vi "example_02_convert.vi"() -> ()   [LabVIEW 2015, in "lv-unit-conversion.lvlib"] (continued)
 gallon per minute foot", "dimension"="L2/T", "is_si_unit"=TRUE, "category"="derived", "base_unit"="m3/(s.m)", "conversion_reference"="DERIVED", "is_exact"=TRUE, "a"=0.0, "b"=0.003785411784, "c"=18.288, "d"=0.0, "underlying_def"="", "description"=""}, {"symbol"="m3/(d.m)", "name"="(cubic metre per day) per metre", "dimension"="L2/T", "is_si_unit"=TRUE, "category"="derived", "base_unit"="m3/(s.m)", "conversion_reference"="DERIVED", "is_exact"=TRUE, "a"=0.0, "b"=1.0, "c"=86400.0, "d"=0.0, "underlying_def"="", "description"=""}, {"symbol"="m3/(h.m)", "name"="(cubic metre per hour) per metre", "dimension"="L2/T", "is_si_unit"=TRUE, "category"="derived", "base_unit"="m3/(s.m)", "conversion_reference"="DERIVED", "is_exact"=TRUE, "a"=0.0, "b"=1.0, "c"=3600.0, "d"=0.0, "underlying_def"="", "description"=""}, {"symbol"="m3/(s.ft)", "name"="(cubic metre per second) per foot", "dimension"="L2/T", "is_si_unit"=TRUE, "category"="derived", "base_unit"="m3/(s.m)", "conversion_reference"="DERIVED", "is_exact"=TRUE, "a"=0.0, "b"=1.0, "c"=0.3048, "d"=0.0, "underlying_def"="", "description"=""}, {"symbol"="cSt", "name"="centistokes", "dimension"="L2/T", "is_si_unit"=TRUE, "category"="prefixed", "base_unit"="m2/s", "conversion_reference"="DERIVED", "is_exact"=TRUE, "a"=0.0, "b"=1e-06, "c"=1.0, "d"=0.0, "underlying_def"="", "description"=""}, {"symbol"="rd", "name"="rad", "dimension"="L2/T2", "is_si_unit"=TRUE, "category"="atom", "base_unit"="Gy", "conversion_reference"="NIST-SI", "is_exact"=TRUE, "a"=0.0, "b"=0.01, "c"=1.0, "d"=0.0, "underlying_def"="1/100 Gy", "description"="A obsolete unit of absorbed radiation dose. \n\t\t\t\tIt was originally defined in CGS units in 1953 as the dose causing 100 ergs of energy to be absorbed \n\t\t\t\tby one gram of matter. \n\t\t\t\tIt has been replaced by the gray in most of the world.\n\t\t\t"}, {"symbol"="Gy", "name"="gray", "dimension"="L2/T2", "is_si_unit"=TRUE, "category"="atom-special", "base_unit"="", "conversion_reference"="", "is_exact"=FALSE, "a"=0.0, "b"=0.0, "c"=0.0, "d"=0.0, "underlying_def"="J/kg", "description"="The absorbed dose when the energy per unit mass imparted to matter by ionizing radiation is 1 J/kg"}, {"symbol"="Sv", "name"="sievert", "dimension"="L2/T2", "is_si_unit"=TRUE, "category"="atom-special", "base_unit"="", "conversion_reference"="", "is_exact"=FALSE, "a"=0.0, "b"=0.0, "c"=0.0, "d"=0.0, "underlying_def"="J/kg", "description"="The dose equivalent when the absorbed dose of ionizing radiation multiplied by the dimensionless \n\t\t\t\tfactors Q (quality factor) and N (product of any of the multiplying factors) stipulated by the \n\t\t\t\tInternational Commission on Radiological Protection is 1.0 J/kg.\n\t\t\t"}, {"symbol"="rem", "name"="rem", "dimension"="L2/T2", "is_si_unit"=TRUE, "category"="atom-allowed", "base_unit"="Sv", "conversion_reference"="NIST-SI", "is_exact"=TRUE, "a"=0.0, "b"=0.01, "c"=1.0, "d"=0.0, "underlying_def"="1/100 Sv", "description"="A unit of radiation dosage (such as from X rays) applied to humans. \n\t\t\t\tDerived from the phrase Roentgen equivalent man, the rem is now defined as the dosage in rads that \n\t\t\t\twill cause the same amount of biological injury as one rad of X rays or gamma rays.\n\t\t\t"}, {"symbol"="J/kg", "name"="joule per kilogram", "dimension"="L2/T2", "is_si_unit"=TRUE, "category"="derived", "base_unit"="", "conversion_reference"="", "is_exact"=FALSE, "a"=0.0, "b"=0.0, "c"=0.0, "d"=0.0, "underlying_def"="", "description"=""}, {"symbol"="Btu[IT]/lbm", "name"="BTU per pound-mass", "dimension"="L2/T2", "is_si_unit"=TRUE, "category"="derived", "base_unit"="J/kg", "conversion_reference"="DERIVED", "is_exact"=TRUE, "a"=0.0, "b"=2326.0, "c"=1.0, "d"=0.0, "underlying_def"="", "description"=""}, {"symbol"="cal[th]/g", "name"="calorie per gram", "dimension"="L2/T2", "is_si_unit"=TRUE, "category"="derived", "base_unit"="J/kg", "conversion_reference"="DERIVED", "is_exact"=TRUE, "a"=0.0, "b"=4184.0, "c"=1.0, "d"=0.0, "underlying_def"="", "description"=""}, {"symbol"="cal[th]/kg", "name"="calorie per kilogram", "dimension"="L2/T2", "is_si_unit"=TRUE, "category"="derived", "base_unit"="J/kg", "conversion_reference"="DERIVED", "is_exact"=TRUE, "a"=0.0, "b"=4.184, "c"=1.0, "d"=0.0, "underlying_def"="", "description"=""}, {"symbol"="cal[th]/lbm", "name"="calorie per pound-mass", "dimension"="L2/T2", "is_si_unit"=TRUE, "category"="derived", "base_unit"="J/kg", "conversion_reference"="DERIVED", "is_exact"=TRUE, "a"=0.0, "b"=4.184, "c"=0.45359237, "d"=0.0, "underlying_def"="", "description"=""}, {"symbol"="erg/g", "name"="erg per gram", "dimension"="L2/T2", "is_si_unit"=TRUE, "category"="derived", "base_unit"="J/kg", "conversion_reference"="DERIVED", "is_exact"=TRUE, "a"=0.0, "b"=0.0001, "c"=1.0, "d"=0.0, "underlying_def"="", "description"=""}, {"symbol"="erg/kg", "name"="erg per kilogram", "dimension"="L2/T2", "is_si_unit"=TRUE, "category"="derived", "base_unit"="J/kg", "conversion_reference"="DERIVED", "is_exact"=TRUE, "a"=0.0, "b"=1e-07, "c"=1.0, "d"=0.0, "underlying_def"="", "description"=""}, {"symbol"="hp.h/lbm", "name"="horsepower hour per pound-mass", "dimension"="L2/T2", "is_si_unit"=TRUE, "category"="derived", "base_unit"="J/kg", "conversion_reference"="DERIVED", "is_exact"=TRUE, "a"=0.0, "b"=2684519.537696173, "c"=0.45359237, "d"=0.0, "underlying_def"="", "description"=""}, {"symbol"="J/g", "name"="joule per gram", "dimension"="L2/T2", "is_si_unit"=TRUE, "category"="derived", "base_unit"="J/kg", "conversion_reference"="DERIVED", "is_exact"=TRUE, "a"=0.0, "b"=1000.0, "c"=1.0, "d"=0.0, "underlying_def"="", "description"=""}, {"symbol"="kcal[th]/g", "name"="thousand calorie per gram", "dimension"="L2/T2", "is_si_unit"=TRUE, "category"="derived", "base_unit"="J/kg", "conversion_reference"="DERIVED", "is_exact"=TRUE, "a"=0.0, "b"=4184000.0, "c"=1.0, "d"=0.0, "underlying_def"="", "description"=""}, {"symbol"="kcal[th]/kg", "name"="thousand calorie per kilogram", "dimension"="L2/T2", "is_si_unit"=TRUE, "category"="derived", "base_unit"="J/kg", "conversion_reference"="DERIVED", "is_exact"=TRUE, "a"=0.0, "b"=4184.0, "c"=1.0, "d"=0.0, "underlying_def"="", "description"=""}, {"symbol"="kJ/kg", "name"="kilojoule per kilogram", "dimension"="L2/T2", "is_si_unit"=TRUE, "category"="derived", "base_unit"="J/kg", "conversion_reference"="DERIVED", "is_exact"=TRUE, "a"=0.0, "b"=1000.0, "c"=1.0, "d"=0.0, "underlying_def"="", "description"=""}, {"symbol"="kW.h/kg", "name"="kilowatt hour per kilogram", "dimension"="L2/T2", "is_si_unit"=TRUE, "category"="derived", "base_unit"="J/kg", "conversion_reference"="DERIVED", "is_exact"=TRUE, "a"=0.0, "b"=3600000.0, "c"=1.0, "d"=0.0, "underlying_def"="", "description"=""}, {"symbol"="lbf.ft/lbm", "name"="foot pound-force per pound-mass", "dimension"="L2/T2", "is_si_unit"=TRUE, "category"="derived", "base_unit"="J/kg", "conversion_reference"="DERIVED", "is_exact"=TRUE, "a"=0.0, "b"=1.3558179483314003, "c"=0.45359237, "d"=0.0, "underlying_def"="", "description"=""}, {"symbol"="MJ/kg", "name"="megajoule per kilogram", "dimension"="L2/T2", "is_si_unit"=TRUE, "category"="derived", "base_unit"="J/kg", "conversion_reference"="DERIVED", "is_exact"=TRUE, "a"=0.0, "b"=1000000.0, "c"=1.0, "d"=0.0, "underlying_def"="", "description"=""}, {"symbol"="MW.h/kg", "name"="megawatt hour per kilogram", "dimension"="L2/T2", "is_si_unit"=TRUE, "category"="derived", "base_unit"="J/kg", "conversion_reference"="DERIVED", "is_exact"=TRUE, "a"=0.0, "b"=3600000000.0, "c"=1.0, "d"=0.0, "underlying_def"="", "description"=""}, {"symbol"="cGy", "name"="centigray", "dimension"="L2/T2", "is_si_unit"=TRUE, "category"="prefixed", "base_unit"="Gy", "conversion_reference"="DERIVED", "is_exact"=TRUE, "a"=0.0, "b"=0.01, "c"=1.0, "d"=0.0, "underlying_def"="", "description"=""}, {"symbol"="crd", "name"="hundredth of rad", "dimension"="L2/T2", "is_si_unit"=TRUE, "category"="prefixed", "base_unit"="Gy", "conversion_reference"="DERIVED", "is_exact"=TRUE, "a"=0.0, "b"=0.0001, "c"=1.0, "d"=0.0, "underlying_def"="", "description"=""}, {"symbol"="dGy", "name"="decigray", "dimension"="L2/T2", "is_si_unit"=TRUE, "category"="prefixed", "base_unit"="Gy", "conversion_reference"="DERIVED", "is_exact"=TRUE, "a"=0.0, "b"=0.1, "c"=1.0, "d"=0.0, "underlying_def"="", "description"=""}, {"symbol"="drd", "name"="tenth of rad", "dimension"="L2/T2", "is_si_unit"=TRUE, "category"="prefixed", "base_unit"="Gy", "conversion_reference"="DERIVED", "is_exact"=TRUE, "a"=0.0, "b"=0.001, "c"=1.0, "d"=0.0, "underlying_def"="", "description"=""}, {"symbol"="EGy", "name"="exagray", "dimension"="L2/T2", "is_si_unit"=TRUE, "category"="prefixed", "base_unit"="Gy", "conversion_reference"="DERIVED", "is_exact"=TRUE, "a"=0.0, "b"=1e+18, "c"=1.0, "d"=0.0, "underlying_def"="", "description"=""}, {"symbol"="Erd", "name"="million million million rad", "dimension"="L2/T2", "is_si_unit"=TRUE, "category"="prefixed", "base_unit"="Gy", "conversion_reference"="DERIVED", "is_exact"=TRUE, "a"=0.0, "b"=1e+16, "c"=1.0, "d"=0.0, "underlying_def"="", "description"=""}, {"symbol"="fGy", "name"="femtogray", "dimension"="L2/T2", "is_si_unit"=TRUE, "category"="prefixed", "base_unit"="Gy", "conversion_reference"="DERIVED", "is_exact"=TRUE, "a"=0.0, "b"=1e-15, "c"=1.0, "d"=0.0, "underlying_def"="", "description"=""}, {"symbol"="frd", "name"="femtorad", "dimension"="L2/T2", "is_si_unit"=TRUE, "category"="prefixed", "base_unit"="Gy", "conversion_reference"="DERIVED", "is_exact"=TRUE, "a"=0.0, "b"=1e-17, "c"=1.0, "d"=0.0, "underlying_def"="", "description"=""}, {"symbol"="GGy", "name"="gigagray", "dimension"="L2/T2", "is_si_unit"=TRUE, "category"="prefixed", "base_unit"="Gy", "conversion_reference"="DERIVED", "is_exact"=TRUE, "a"=0.0, "b"=1000000000.0, "c"=1.0, "d"=0.0, "underlying_def"="", "description"=""}, {"symbol"="Grd", "name"="thousand million rad", "dimension"="L2/T2", "is_si_unit"=TRUE, "category"="prefixed", "base_unit"="Gy", "conversion_reference"="DERIVED", "is_exact"=TRUE, "a"=0.0, "b"=10000000.0, "c"=1.0, "d"=0.0, "underlying_def"="", "description"=""}, {"symbol"="kGy", "name"="kilogray", "dimension"="L2/T2", "is_si_unit"=TRUE, "category"="prefixed", "base_unit"="Gy", "conversion_reference"="DERIVED", "is_exact"=TRUE, "a"=0.0, "b"=1000.0, "c"=1.0, "d"=0.0, "underlying_def"="", "description"=""}, {"symbol"="krd", "name"="thousand rad", "dimension"="L2/T2", "is_si_unit"=TRUE, "category"="prefixed", "base_unit"="Gy", "conversion_reference"="DERIVED", "is_exact"=TRUE, "a"=0.0, "b"=10.0, "c"=1.0, "d"=0.0, "underlying_def"="", "description"=""}, {"symbol"="mGy", "name"="milligray", "dimension"="L2/T2", "is_si_unit"=TRUE, "category"="prefixed", "base_unit"="Gy", "conversion_reference"="DERIVED", "is_exact"=TRUE, "a"=0.0, "b"=0.001, "c"=1.0, "d"=0.0, "underlying_def"="", "description"=""}, {"symbol"="MGy", "name"="megagray", "dimension"="L2/T2", "is_si_unit"=TRUE, "category"="prefixed", "base_unit"="Gy", "conversion_reference"="DERIVED", "is_exact"=TRUE, "a"=0.0, "b"=1000000.0, "c"=1.0, "d"=0.0, "underlying_def"="", "description"=""}, {"symbol"="mrd", "name"="thousandth of rad", "dimension"="L2/T2", "is_si_unit"=TRUE, "category"="prefixed", "base_unit"="Gy", "conversion_reference"="DERIVED", "is_exact"=TRUE, "a"=0.0, "b"=1e-05, "c"=1.0, "d"=0.0, "underlying_def"="", "description"=""}, {"symbol"="Mrd", "name"="million rad", "dimension"="L2/T2", "is_si_unit"=TRUE, "category"="prefixed", "base_unit"="Gy", "conversion_reference"="DERIVED", "is_exact"=TRUE, "a"=0.0, "b"=10000.0, "c"=1.0, "d"=0.0, "underlying_def"="", "description"=""}, {"symbol"="nGy", "name"="nanogray", "dimension"="L2/T2", "is_si_unit"=TRUE, "category"="prefixed", "base_unit"="Gy", "conversion_reference"="DERIVED", "is_exact"=TRUE, "a"=0.0, "b"=1e-09, "c"=1.0, "d"=0.0, "underlying_def"="", "description"=""}, {"symbol"="nrd", "name"="nanorad", "dimension"="L2/T2", "is_si_unit"=TRUE, "category"="prefixed", "base_unit"="Gy", "conversion_reference"="DERIVED", "is_exact"=TRUE, "a"=0.0, "b"=1e-11, "c"=1.0, "d"=0.0, "underlying_def"="", "description"=""}, {"symbol"="pGy", "name"="picogray", "dimension"="L2/T2", "is_si_unit"=TRUE, "category"="prefixed", "base_unit"="Gy", "conversion_reference"="DERIVED", "is_exact"=TRUE, "a"=0.0, "b"=1e-12, "c"=1.0, "d"=0.0, "underlying_def"="", "description"=""}, {"symbol"="prd", "name"="picorad", "dimension"="L2/T2", "is_si_unit"=TRUE, "category"="prefixed", "base_unit"="Gy", "conversion_reference"="DERIVED", "is_exact"=TRUE, "a"=0.0, "b"=1e-14, "c"=1.0, "d"=0.0, "underlying_def"="", "description"=""}, {"symbol"="TGy", "name"="teragray", "dimension"="L2/T2", "is_si_unit"=TRUE, "category"="prefixed", "base_unit"="Gy", "conversion_reference"="DERIVED", "is_exact"=TRUE, "a"=0.0, "b"=1000000000000.0, "c"=1.0, "d"=0.0, "underlying_def"="", "description"=""}, {"symbol"="Trd", "name"="million million rad", "dimension"="L2/T2", "is_si_unit"=TRUE, "category"="prefixed", "base_unit"="Gy", "conversion_reference"="DERIVED", "is_exact"=TRUE, "a"=0.0, "b"=10000000000.0, "c"=1.0, "d"=0.0, "underlying_def"="", "description"=""}, {"symbol"="uGy", "name"="microgray", "dimension"="L2/T2", "is_si_unit"=TRUE, "category"="prefixed", "base_unit"="Gy", "conversion_reference"="DERIVED", "is_exact"=TRUE, "a"=0.0, "b"=1e-06, "c"=1.0, "d"=0.0, "underlying_def"="", "description"=""}, {"symbol"="urd", "name"="millionth of rad", "dimension"="L2/T2", "is_si_unit"=TRUE, "category"="prefixed", "base_unit"="Gy", "conversion_reference"="DERIVED", "is_exact"=TRUE, "a"=0.0, "b"=1e-08, "c"=1.0, "d"=0.0, "underlying_def"="", "description"=""}, {"symbol"="mrem", "name"="thousandth of rem", "dimension"="L2/T2", "is_si_unit"=TRUE, "category"="prefixed", "base_unit"="Sv", "conversion_reference"="DERIVED", "is_exact"=TRUE, "a"=0.0, "b"=1e-05, "c"=1.0, "d"=0.0, "underlying_def"="", "description"=""}, {"symbol"="mSv", "name"="millisievert", "dimension"="L2/T2", "is_si_unit"=TRUE, "category"="prefixed", "base_unit"="Sv", "conversion_reference"="DERIVED", "is_exact"=TRUE, "a"=0.0, "b"=0.001, "c"=1.0, "d"=0.0, "underlying_def"="", "description"=""}, {"symbol"="Sv/s", "name"="sievert per second", "dimension"="L2/T3", "is_si_unit"=TRUE, "category"="derived", "base_unit"="", "conversion_reference"="", "is_exact"=FALSE, "a"=0.0, "b"=0.0, "c"=0.0, "d"=0.0, "underlying_def"="", "description"="The dose equivalent rate when the absorbed dose per second of ionizing radiation multiplied by the \n\t\t\t\tappropriate factors is equivalent to 1 Sievert per second.\n\t\t\t"}, {"symbol"="mrem/h", "name"="thousandth of irem per hour", "dimension"="L2/T3", "is_si_unit"=TRUE, "category"="derived", "base_unit"="Sv/s", "conversion_reference"="DERIVED", "is_exact"=TRUE, "a"=0.0, "b"=1e-05, "c"=3600.0, "d"=0.0, "underlying_def"="", "description"=""}, {"symbol"="mSv/h", "name"="millisievert per hour", "dimension"="L2/T3", "is_si_unit"=TRUE, "category"="derived", "base_unit"="Sv/s", "conversion_reference"="DERIVED", "is_exact"=TRUE, "a"=0.0, "b"=0.001, "c"=3600.0, "d"=0.0, "underlying_def"="", "description"=""}, {"symbol"="rem/h", "name"="rem per hour", "dimension"="L2/T3", "is_si_unit"=TRUE, "category"="derived", "base_unit"="Sv/s", "conversion_reference"="DERIVED", "is_exact"=TRUE, "a"=0.0, "b"=0.01, "c"=3600.0, "d"=0.0, "underlying_def"="", "description"=""}, {"symbol"="Sv/h", "name"="sievert per hour", "dimension"="L2/T3", "is_si_unit"=TRUE, "category"="derived", "base_unit"="Sv/s", "conversion_reference"="DERIVED", "is_exact"=TRUE, "a"=0.0, "b"=1.0, "c"=3600.0, "d"=0.0, "underlying_def"="", "description"=""}, {"symbol"="kg.m2", "name"="kilogram square metre", "dimension"="L2M", "is_si_unit"=TRUE, "category"="derived", "base_unit"="", "conversion_reference"="", "is_exact"=FALSE, "a"=0.0, "b"=0.0, "c"=0.0, "d"=0.0, "underlying_def"="", "description"=""}, {"symbol"="lbm.ft2", "name"="pound-mass square foot", "dimension"="L2M", "is_si_unit"=TRUE, "category"="derived", "base_unit"="kg.m2", "conversion_reference"="DERIVED", "is_exact"=TRUE, "a"=0.0, "b"=0.0421401100938048, "c"=1.0, "d"=0.0, "underlying_def"="", "description"=""}, {"symbol"="J/(mol.deltaK)", "name"="joule per gram-mole delta kelvin", "dimension"="L2M/DNT2", "is_si_unit"=TRUE, "category"="derived", "base_unit"="", "conversion_reference"="", "is_exact"=FALSE, "a"=0.0, "b"=0.0, "c"=0.0, "d"=0.0, "underlying_def"="", "description"=""}, {"symbol"="Btu[IT]/(lbmol.deltaF)", "name"="BTU per pound-mass-mole delta Fahrenheit", "dimension"="L2M/DNT2", "is_si_unit"=TRUE, "category"="derived", "base_unit"="J/(mol.deltaK)", "conversion_reference"="DERIVED", "is_exact"=TRUE, "a"=0.0, "b"=4.1868, "c"=1.0, "d"=0.0, "underlying_def"="", "description"=""}, {"symbol"="cal[th]/(mol.deltaC)", "name"="calorie per gram-mole delta Celsius", "dimension"="L2M/DNT2", "is_si_unit"=TRUE, "category"="derived", "base_unit"="J/(mol.deltaK)", "conversion_reference"="DERIVED", "is_exact"=TRUE, "a"=0.0, "b"=4.184, "c"=1.0, "d"=0.0, "underlying_def"="", "description"=""}, {"symbol"="kJ/(kmol.deltaK)", "name"="kilojoule per kilogram-mole delta kelvin", "dimension"="L2M/DNT2", "is_si_unit"=TRUE, "category"="derived", "base_unit"="J/(mol.deltaK)", "conversion_reference"="DERIVED", "is_exact"=TRUE, "a"=0.0, "b"=1.0, "c"=1.0, "d"=0.0, "underlying_def"="", "description"=""}, {"symbol"="J/deltaK", "name"="joule per delta kelvin", "dimension"="L2M/DT2", "is_si_unit"=TRUE, "category"="derived", "base_unit"="", "conversion_reference"="", "is_exact"=FALSE, "a"=0.0, "b"=0.0, "c"=0.0, "d"=0.0, "underlying_def"="", "description"=""}, {"symbol"="W/deltaK", "name"="watt per delta kelvin", "dimension"="L2M/DT3", "is_si_unit"=TRUE, "category"="derived", "base_unit"="", "conversion_reference"="", "is_exact"=FALSE, "a"=0.0, "b"=0.0, "c"=0.0, "d"=0.0, "underlying_def"="", "description"=""}, {"symbol"="H", "name"="henry", "dimension"="L2M/I2T2", "is_si_unit"=TRUE, "category"="atom-special", "base_unit"="", "conversion_reference"="", "is_exact"=FALSE, "a"=0.0, "b"=0.0, "c"=0.0, "d"=0.0, "underlying_def"="Wb/A", "description"="The inductance of a closed circuit in which an electromotive force of 1 V is produced when the \n\t\t\t\telectric current in the circuit varies uniformly at a rate of 1 A/s.\n\t\t\t"}, {"symbol"="cH", "name"="centihenry", "dimension"="L2M/I2T2", "is_si_unit"=TRUE, "category"="prefixed", "base_unit"="H", "conversion_reference"="DERIVED", "is_exact"=TRUE, "a"=0.0, "b"=0.01, "c"=1.0, "d"=0.0, "underlying_def"="", "description"=""}, {"symbol"="dH", "name"="decihenry", "dimension"="L2M/I2T2", "is_si_unit"=TRUE, "category"="prefixed", "base_unit"="H", "conversion_reference"="DERIVED", "is_exact"=TRUE, "a"=0.0, "b"=0.1, "c"=1.0, "d"=0.0, "underlying_def"="", "description"=""}, {"symbol"="EH", "name"="exahenry", "dimension"="L2M/I2T2", "is_si_unit"=TRUE, "category"="prefixed", "base_unit"="H", "conversion_reference"="DERIVED", "is_exact"=TRUE, "a"=0.0, "b"=1e+18, "c"=1.0, "d"=0.0, "underlying_def"="", "description"=""}, {"symbol"="fH", "name"="femtohenry", "dimension"="L2M/I2T2", "is_si_unit"=TRUE, "category"="prefixed", "base_unit"="H", "conversion_reference"="DERIVED", "is_exact"=TRUE, "a"=0.0, "b"=1e-15, "c"=1.0, "d"=0.0, "underlying_def"="", "description"=""}, {"symbol"="GH", "name"="gigahenry", "dimension"="L2M/I2T2", "is_si_unit"=TRUE, "category"="prefixed", "base_unit"="H", "conversion_reference"="DERIVED", "is_exact"=TRUE, "a"=0.0, "b"=1000000000.0, "c"=1.0, "d"=0.0, "underlying_def"="", "description"=""}, {"symbol"="kH", "name"="kilohenry", "dimension"="L2M/I2T2", "is_si_unit"=TRUE, "category"="prefixed", "base_unit"="H", "conversion_reference"="DERIVED", "is_exact"=TRUE, "a"=0.0, "b"=1000.0, "c"=1.0, "d"=0.0, "underlying_def"="", "description"=""}, {"symbol"="mH", "name"="millihenry", "dimension"="L2M/I2T2", "is_si_unit"=TRUE, "category"="prefixed", "base_unit"="H", "conversion_reference"="DERIVED", "is_exact"=TRUE, "a"=0.0, "b"=0.001, "c"=1.0, "d"=0.0, "underlying_def"="", "description"=""}, {"symbol"="MH", "name"="megahenry", "dimension"="L2M/I2T2", "is_si_unit"=TRUE, "category"="prefixed", "base_unit"="H", "conversion_reference"="DERIVED", "is_exact"=TRUE, "a"=0.0, "b"=1000000.0, "c"=1.0, "d"=0.0, "underlying_def"="", "description"=""}, {"symbol"="nH", "name"="nanohenry", "dimension"="L2M/I2T2", "is_si_unit"=TRUE, "category"="prefixed", "base_unit"="H", "conversion_reference"="DERIVED", "is_exact"=TRUE, "a"=0.0, "b"=1e-09, "c"=1.0, "d"=0.0, "underlying_def"="", "description"=""}, {"symbol"="TH", "name"="terahenry", "dimension"="L2M/I2T2", "is_si_unit"=TRUE, "category"="prefixed", "base_unit"="H", "conversion_reference"="DERIVED", "is_exact"=TRUE, "a"=0.0, "b"=1000000000000.0, "c"=1.0, "d"=0.0, "underlying_def"="", "description"=""}, {"symbol"="uH", "name"="microhenry", "dimension"="L2M/I2T2", "is_si_unit"=TRUE, "category"="prefixed", "base_unit"="H", "conversion_reference"="DERIVED", "is_exact"=TRUE, "a"=0.0, "b"=1e-06, "c"=1.0, "d"=0.0, "underlying_def"="", "description"=""}, {"symbol"="ohm", "name"="ohm", "dimension"="L2M/I2T3", "is_si_unit"=TRUE, "category"="atom-special", "base_unit"="", "conversion_reference"="", "is_exact"=FALSE, "a"=0.0, "b"=0.0, "c"=0.0, "d"=0.0, "underlying_def"="V/A", "description"="The electric resistance between two points of a conductor when a constant difference of potential of \n\t\t\t\t1 V, applied between these two points, produces in this conductor a current of 1 A, this conductor \n\t\t\t\tnot being the source of any electromotive force.\n\t\t\t"}, {"symbol"="cohm", "name"="centiohm", "dimension"="L2M/I2T3", "is_si_unit"=TRUE, "category"="prefixed", "base_unit"="ohm", "conversion_reference"="DERIVED", "is_exact"=TRUE, "a"=0.0, "b"=0.01, "c"=1.0, "d"=0.0, "underlying_def"="", "description"=""}, {"symbol"="dohm", "name"="deciohm", "dimension"="L2M/I2T3", "is_si_unit"=TRUE, "category"="prefixed", "base_unit"="ohm", "conversion_reference"="DERIVED", "is_exact"=TRUE, "a"=0.0, "b"=0.1, "c"=1.0, "d"=0.0, "underlying_def"="", "description"=""}, {"symbol"="Eohm", "name"="exaohm", "dimension"="L2M/I2T3", "is_si_unit"=TRUE, "category"="prefixed", "base_unit"="ohm", "conversion_reference"="DERIVED", "is_exact"=TRUE, "a"=0.0, "b"=1e+18, "c"=1.0, "d"=0.0, "underlying_def"="", "description"=""}, {"symbol"="fohm", "name"="femtoohm", "dimension"="L2M/I2T3", "is_si_unit"=TRUE, "category"="prefixed", "base_unit"="ohm", "conversion_reference"="DERIVED", "is_exact"=TRUE, "a"=0.0, "b"=1e-15, "c"=1.0, "d"=0.0, "underlying_def"="", "description"=""}, {"symbol"="Gohm", "name"="gigaohm", "dimension"="L2M/I2T3", "is_si_unit"=TRUE, "category"="prefixed", "base_unit"="ohm", "conversion_reference"="DERIVED", "is_exact"=TRUE, "a"=0.0, "b"=1000000000.0, "c"=1.0, "d"=0.0, "underlying_def"="", "description"=""}, {"symbol"="kohm", "name"="kilohm", "dimension"="L2M/I2T3", "is_si_unit"=TRUE, "category"="prefixed", "base_unit"="ohm", "conversion_reference"="DERIVED", "is_exact"=TRUE, "a"=0.0, "b"=1000.0, "c"=1.0, "d"=0.0, "underlying_def"="", "description"=""}, {"symbol"="mohm", "name"="milliohm", "dimension"="L2M/I2T3", "is_si_unit"=TRUE, "category"="prefixed", "base_unit"="ohm", "conversion_reference"="DERIVED", "is_exact"=TRUE, "a"=0.0, "b"=0.001, "c"=1.0, "d"=0.0, "underlying_def"="", "description"=""}, {"symbol"="Mohm", "name"="megohm", "dimension"="L2M/I2T3", "is_si_unit"=TRUE, "category"="prefixed", "base_unit"="ohm", "conversion_reference"="DERIVED", "is_exact"=TRUE, "a"=0.0, "b"=1000000.0, "c"=1.0, "d"=0.0, "underlying_def"="", "description"=""}, {"symbol"="nohm", "name"="nanoohm", "dimension"="L2M/I2T3", "is_si_unit"=TRUE, "category"="prefixed", "base_unit"="ohm", "conversion_reference"="DERIVED", "is_exact"=TRUE, "a"=0.0, "b"=1e-09, "c"=1.0, "d"=0.0, "underlying_def"="", "description"=""}, {"symbol"="pohm", "name"="picoohm", "dimension"="L2M/I2T3", "is_si_unit"=TRUE, "category"="prefixed", "base_unit"="ohm", "conversion_reference"="DERIVED", "is_exact"=TRUE, "a"=0.0, "b"=1e-12, "c"=1.0, "d"=0.0, "underlying_def"="", "description"=""}, {"symbol"="Tohm", "name"="teraohm", "dimension"="L2M/I2T3", "is_si_unit"=TRUE, "category"="prefixed", "base_unit"="ohm", "conversion_reference"="DERIVED", "is_exact"=TRUE, "a"=0.0, "b"=1000000000000.0, "c"=1.0, "d"=0.0, "underlying_def"="", "description"=""}, {"symbol"="uohm", "name"="microohm", "dimension"="L2M/I2T3", "is_si_unit"=TRUE, "category"="prefixed", "base_unit"="ohm", "conversion_reference"="DERIVED", "is_exact"=TRUE, "a"=0.0, "b"=1e-06, "c"=1.0, "d"=0.0, "underlying_def"="", "description"=""}, {"symbol"="Wb", "name"="weber", "dimension"="L2M/IT2", "is_si_unit"=TRUE, "category"="atom-special", "base_unit"="", "conversion_reference"="", "is_exact"=FALSE, "a"=0.0, "b"=0.0, "c"=0.0, "d"=0.0, "underlying_def"="V.s", "description"="The magnetic flux which, linking a circuit of one turn, produces in it an electromotive force of 1 V \n\t\t\t\tas it is reduced to zero at a uniform rate in 1 s.\n\t\t\t"}, {"symbol"="cWb", "name"="centiweber", "dimension"="L2M/IT2", "is_si_unit"=TRUE, "category"="prefixed", "base_unit"="Wb", "conversion_reference"="DERIVED", "is_exact"=TRUE, "a"=0.0, "b"=0.01, "c"=1.0, "d"=0.0, "underlying_def"="", "description"=""}, {"symbol"="dWb", "name"="deciweber", "dimension"="L2M/IT2", "is_si_unit"=TRUE, "category"="prefixed", "base_unit"="Wb", "conversion_reference"="DERIVED", "is_exact"=TRUE, "a"=0.0, "b"=0.1, "c"=1.0, "d"=0.0, "underlying_def"="", "description"=""}, {"symbol"="EWb", "name"="exaweber", "dimension"="L2M/IT2", "is_si_unit"=TRUE, "category"="prefixed", "base_unit"="Wb", "conversion_reference"="DERIVED", "is_exact"=TRUE, "a"=0.0, "b"=1e+18, "c"=1.0, "d"=0.0, "underlying_def"="", "description"=""}, {"symbol"="fWb", "name"="femtoweber", "dimension"="L2M/IT2", "is_si_unit"=TRUE, "category"="prefixed", "base_unit"="Wb", "conversion_reference"="DERIVED", "is_exact"=TRUE, "a"=0.0, "b"=1e-15, "c"=1.0, "d"=0.0, "underlying_def"="", "description"=""}, {"symbol"="GWb", "name"="gigaweber", "dimension"="L2M/IT2", "is_si_unit"=TRUE, "category"="prefixed", "base_unit"="Wb", "conversion_reference"="DERIVED", "is_exact"=TRUE, "a"=0.0, "b"=1000000000.0, "c"=1.0, "d"=0.0, "underlying_def"="", "description"=""}, {"symbol"="kWb", "name"="kiloweber", "dimension"="L2M/IT2", "is_si_unit"=TRUE, "category"="prefixed", "base_unit"="Wb", "conversion_reference"="DERIVED", "is_exact"=TRUE, "a"=0.0, "b"=1000.0, "c"=1.0, "d"=0.0, "underlying_def"="", "description"=""}, {"symbol"="mWb", "name"="milliweber", "dimension"="L2M/IT2", "is_si_unit"=TRUE, "category"="prefixed", "base_unit"="Wb", "conversion_reference"="DERIVED", "is_exact"=TRUE, "a"=0.0, "b"=0.001, "c"=1.0, "d"=0.0, "underlying_def"="", "description"=""}, {"symbol"="MWb", "name"="megaweber", "dimension"="L2M/IT2", "is_si_unit"=TRUE, "category"="prefixed", "base_unit"="Wb", "conversion_reference"="DERIVED", "is_exact"=TRUE, "a"=0.0, "b"=1000000.0, "c"=1.0, "d"=0.0, "underlying_def"="", "description"=""}, {"symbol"="nWb", "name"="nanoweber", "dimension"="L2M/IT2", "is_si_unit"=TRUE, "category"="prefixed", "base_unit"="Wb", "conversion_reference"="DERIVED", "is_exact"=TRUE, "a"=0.0, "b"=1e-09, "c"=1.0, "d"=0.0, "underlying_def"="", "description"=""}, {"symbol"="pWb", "name"="picoweber", "dimension"="L2M/IT2", "is_si_unit"=TRUE, "category"="prefixed", "base_unit"="Wb", "conversion_reference"="DERIVED", "is_exact"=TRUE, "a"=0.0, "b"=1e-12, "c"=1.0, "d"=0.0, "underlying_def"="", "description"=""}, {"symbol"="TWb", "name"="teraweber", "dimension"="L2M/IT2", "is_si_unit"=TRUE, "category"="prefixed", "base_unit"="Wb", "conversion_reference"="DERIVED", "is_exact"=TRUE, "a"=0.0, "b"=1000000000000.0, "c"=1.0, "d"=0.0, "underlying_def"="", "description"=""}, {"symbol"="uWb", "name"="microweber", "dimension"="L2M/IT2", "is_si_unit"=TRUE, "category"="prefixed", "base_unit"="Wb", "conversion_reference"="DERIVED", "is_exact"=TRUE, "a"=0.0, "b"=1e-06, "c"=1.0, "d"=0.0, "underlying_def"="", "description"=""}, {"symbol"="V", "name"="volt", "dimension"="L2M/IT3", "is_si_unit"=TRUE, "category"="atom-special", "base_unit"="", "conversion_reference"="", "is_exact"=FALSE, "a"=0.0, "b"=0.0, "c"=0.0, "d"=0.0, "underlying_def"="W/A", "description"="The difference of electric potential between two points of a conductor carrying a constant current \n\t\t\t\tof 1 A when the power dissipated between these points is equal to 1 W.\n\t\t\t"}, {"symbol"="cV", "name"="centivolt", "dimension"="L2M/IT3", "is_si_unit"=TRUE, "category"="prefixed", "base_unit"="V", "conversion_reference"="DERIVED", "is_exact"=TRUE, "a"=0.0, "b"=0.01, "c"=1.0, "d"=0.0, "underlying_def"="", "description"=""}, {"symbol"="dV", "name"="decivolt", "dimension"="L2M/IT3", "is_si_unit"=TRUE, "category"="prefixed", "base_unit"="V", "conversion_reference"="DERIVED", "is_exact"=TRUE, "a"=0.0, "b"=0.1, "c"=1.0, "d"=0.0, "underlying_def"="", "description"=""}, {"symbol"="fV", "name"="femtovolt", "dimension"="L2M/IT3", "is_si_unit"=TRUE, "category"="prefixed", "base_unit"="V", "conversion_reference"="DERIVED", "is_exact"=TRUE, "a"=0.0, "b"=1e-15, "c"=1.0, "d"=0.0, "underlying_def"="", "description"=""}, {"symbol"="GV", "name"="gigavolt", "dimension"="L2M/IT3", "is_si_unit"=TRUE, "category"="prefixed", "base_unit"="V", "conversion_reference"="DERIVED", "is_exact"=TRUE, "a"=0.0, "b"=1000000000.0, "c"=1.0, "d"=0.0, "underlying_def"="", "description"=""}, {"symbol"="kV", "name"="kilovolt", "dimension"="L2M/IT3", "is_si_unit"=TRUE, "category"="prefixed", "base_unit"="V", "conversion_reference"="DERIVED", "is_exact"=TRUE, "a"=0.0, "b"=1000.0, "c"=1.0, "d"=0.0, "underlying_def"="", "description"=""}, {"symbol"="mV", "name"="millivolt", "dimension"="L2M/IT3", "is_si_unit"=TRUE, "category"="prefixed", "base_unit"="V", "conversion_reference"="DERIVED", "is_exact"=TRUE, "a"=0.0, "b"=0.001, "c"=1.0, "d"=0.0, "underlying_def"="", "description"=""}, {"symbol"="MV", "name"="megavolt", "dimension"="L2M/IT3", "is_si_unit"=TRUE, "category"="prefixed", "base_unit"="V", "conversion_reference"="DERIVED", "is_exact"=TRUE, "a"=0.0, "b"=1000000.0, "c"=1.0, "d"=0.0, "underlying_def"="", "description"=""}, {"symbol"="nV", "name"="nanovolt", "dimension"="L2M/IT3", "is_si_unit"=TRUE, "category"="prefixed", "base_unit"="V", "conversion_reference"="DERIVED", "is_exact"=TRUE, "a"=0.0, "b"=1e-09, "c"=1.0, "d"=0.0, "underlying_def"="", "description"=""}, {"symbol"="pV", "name"="picovolt", "dimension"="L2M/IT3", "is_si_unit"=TRUE, "category"="prefixed", "base_unit"="V", "conversion_reference"="DERIVED", "is_exact"=TRUE, "a"=0.0, "b"=1e-12, "c"=1.0, "d"=0.0, "underlying_def"="", "description"=""}, {"symbol"="TV", "name"="teravolt", "dimension"="L2M/IT3", "is_si_unit"=TRUE, "category"="prefixed", "base_unit"="V", "conversion_reference"="DERIVED", "is_exact"=TRUE, "a"=0.0, "b"=1000000000000.0, "c"=1.0, "d"=0.0, "underlying_def"="", "description"=""}, {"symbol"="uV", "name"="microvolt", "dimension"="L2M/IT3", "is_si_unit"=TRUE, "category"="prefixed", "base_unit"="V", "conversion_reference"="DERIVED", "is_exact"=TRUE, "a"=0.0, "b"=1e-06, "c"=1.0, "d"=0.0, "underlying_def"="", "description"=""}, {"symbol"="J/mol", "name"="joule per gram-mole", "dimension"="L2M/NT2", "is_si_unit"=TRUE, "category"="derived", "base_unit"="", "conversion_reference"="", "is_exact"=FALSE, "a"=0.0, "b"=0.0, "c"=0.0, "d"=0.0, "underlying_def"="", "description"=""}, {"symbol"="Btu[IT]/lbmol", "name"="BTU per pound-mass-mole", "dimension"="L2M/NT2", "is_si_unit"=TRUE, "category"="derived", "base_unit"="J/mol", "conversion_reference"="DERIVED", "is_exact"=TRUE, "a"=0.0, "b"=2.326, "c"=1.0, "d"=0.0, "underlying_def"="", "description"=""}, {"symbol"="kcal[th]/mol", "name"="thousand calorie per gram-mole", "dimension"="L2M/NT2", "is_si_unit"=TRUE, "category"="derived", "base_unit"="J/mol", "conversion_reference"="DERIVED", "is_exact"=TRUE, "a"=0.0, "b"=4184.0, "c"=1.0, "d"=0.0, "underlying_def"="", "description"=""}, {"symbol"="kJ/kmol", "name"="kilojoule per kilogram-mole", "dimension"="L2M/NT2", "is_si_unit"=TRUE, "category"="derived", "base_unit"="J/mol", "conversion_reference"="DERIVED", "is_exact"=TRUE, "a"=0.0, "b"=1.0, "c"=1.0, "d"=0.0, "underlying_def"="", "description"=""}, {"symbol"="MJ/kmol", "name"="megajoule per kilogram-mole", "dimension"="L2M/NT2", "is_si_unit"=TRUE, "category"="derived", "base_unit"="J/mol", "conversion_reference"="DERIVED", "is_exact"=TRUE, "a"=0.0, "b"=1000.0, "c"=1.0, "d"=0.0, "underlying_def"="", "description"=""}, {"symbol"="W/sr", "name"="watt per steradian", "dimension"="L2M/ST3", "is_si_unit"=TRUE, "category"="derived", "base_unit"="", "conversion_reference"="", "is_exact"=FALSE, "a"=0.0, "b"=0.0, "c"=0.0, "d"=0.0, "underlying_def"="", "description"=""}, {"symbol"="J", "name"="joule", "dimension"="L2M/T2", "is_si_unit"=TRUE, "category"="atom-special", "base_unit"="", "conversion_reference"="", "is_exact"=FALSE, "a"=0.0, "b"=0.0, "c"=0.0, "d"=0.0, "underlying_def"="N.m", "description"="The work done when the point of application of a force of 1 N is displaced a distance of 1 m in the \n\t\t\t\tdirection of the force.\n\t\t\t"}, {"symbol"="Btu[IT]", "name"="British thermal unit", "dimension"="L2M/T2", "is_si_unit"=TRUE, "category"="atom", "base_unit"="J", "conversion_reference"="NIST-SI", "is_exact"=TRUE, "a"=0.0, "b"=1055.05585262, "c"=1.0, "d"=0.0, "underlying_def"="", "description"="The amount of heat required to raise the temperature of 1 pound-mass of water 1 degree Fahrenheit. \n\t\t\t\tUses the International Table (IT) calorie which was defined by the Fifth International Conference on \n\t\t\t\tthe Properties of Steam (London, July 1956) to be exactly 4.1868 J. \n\t\t\t\tIn order to convert from calorie to BTU, multiply by the conversion from gram to pound-mass and \n\t\t\t\tmultiply by the conversion from Celsius interval to Fahrenheit interval. \n\t\t\t\tThat is, 1 calorie= (1e-3/ 0.45359237)*(1/(5/9)) BTU= (.001*9)/(5*0.45359237) BTU= (9/2.26796185e+3) \n\t\t\t\tBTU. \n\t\t\t\tGiven, cal[IT]=4.1868 J, it follows that Btu[IT] = (4.1868*2.26796185e+3)/9 = 1,055.05585262 J.\n\t\t\t"}, {"symbol"="Btu[th]", "name"="thermochemical British thermal unit", "dimension"="L2M/T2", "is_si_unit"=TRUE, "category"="atom", "base_unit"="J", "conversion_reference"="DEFINITION", "is_exact"=TRUE, "a"=0.0, "b"=9489.1523804, "c"=9.0, "d"=0.0, "underlying_def"="", "description"="The amount of heat required to raise the temperature of 1 pound-mass of water 1 degree Fahrenheit. \n\t\t\t\tBased on the thermochemical calorie. \n\t\t\t\tIn order to convert from calorie to BTU, multiply by the conversion from gram to pound-mass and \n\t\t\t\tmultiply by the conversion from Celsius interval to Fahrenheit interval. \n\t\t\t\tThat is, calorie = (1e-3/ 0.45359237)*(1/(5/9)) BTU = (.001*9)/(5*0.45359237) BTU = \n\t\t\t\t(9/2.26796185e+3) BTU. \n\t\t\t\tGiven, cal[th] = 4.184 J, it follows that Btu[th] = (4.184*2.26796185e+3)/9 J = (9.4891523804e+3)/9 \n\t\t\t\tJ which is approximately 1.0543502644888888888888888888889e+3 J.\n\t\t\t"}, {"symbol"="Btu[UK]", "name"="United Kingdom British thermal unit", "dimension"="L2M/T2", "is_si_unit"=TRUE, "category"="atom", "base_unit"="J", "conversion_reference"="UK-1995", "is_exact"=TRUE, "a"=0.0, "b"=1055.05585257348, "c"=1.0, "d"=0.0, "underlying_def"="", "description"="The legal unit used in the United Kingdom."}, {"symbol"="cal[IT]", "name"="calorie [International Table]", "dimension"="L2M/T2", "is_si_unit"=TRUE, "category"="atom", "base_unit"="J", "conversion_reference"="NIST-SI", "is_exact"=TRUE, "a"=0.0, "b"=4.1868, "c"=1.0, "d"=0.0, "underlying_def"="", "description"="This uses the International Table definition. \n\t\t\t\tThe amount of heat required at a pressure of one atmosphere to raise the temperature of one gram of \n\t\t\t\twater one degree Celsius.\n\t\t\t"}, {"symbol"="cal[th]", "name"="calorie", "dimension"="L2M/T2", "is_si_unit"=TRUE, "category"="atom", "base_unit"="J", "conversion_reference"="NIST-SI", "is_exact"=TRUE, "a"=0.0, "b"=4.184, "c"=1.0, "d"=0.0, "underlying_def"="", "description"="This uses the thermochemical definition. \n\t\t\t\tThe amount of heat required at a pressure of one atmosphere to raise the temperature of one gram of \n\t\t\t\twater one degree Celsius.\n\t\t\t"}, {"symbol"="erg", "name"="erg", "dimension"="L2M/T2", "is_si_unit"=TRUE, "category"="atom", "base_unit"="J", "conversion_reference"="NIST-SI", "is_exact"=TRUE, "a"=0.0, "b"=1e-07, "c"=1.0, "d"=0.0, "underlying_def"="dyne.cm", "description"="An erg is the amount of work done by a force of one dyne exerted for a distance of one centimeter."}, {"symbol"="eV", "name"="electronvolt", "dimension"="L2M/T2", "is_si_unit"=TRUE, "category"="atom-allowed", "base_unit"="J", "conversion_reference"="NIST-SI", "is_exact"=TRUE, "a"=0.0, "b"=1.602176487e-19, "c"=1.0, "d"=0.0, "underlying_def"="", "description"="The electronvolt is the kinetic energy acquired by an electron in passing through a potential \n\t\t\t\tdifference of 1 V in vacuum, 1.602 176 487(40) x 10-19 J. \n\t\t\t\tThis value of 1 eV is the 2006 CODATA recommended value with the standard uncertainty in the last \n\t\t\t\ttwo digits given in parenthesis. \n\t\t\t\tFrom NIST-SI.\n\t\t\t"}, {"symbol"="quad", "name"="quad", "dimension"="L2M/T2", "is_si_unit"=TRUE, "category"="atom", "base_unit"="J", "conversion_reference"="NIST-SI", "is_exact"=TRUE, "a"=0.0, "b"=1.05505585262e+18, "c"=1.0, "d"=0.0, "underlying_def"="1e15 Btu[IT]", "description"="A quad is a unit of energy equal to 1E+15 (international table) BTU."}, {"symbol"="therm[EC]", "name"="European Community therm", "dimension"="L2M/T2", "is_si_unit"=TRUE, "category"="atom", "base_unit"="J", "conversion_reference"="NIST-SI", "is_exact"=TRUE, "a"=0.0, "b"=105506000.0, "c"=1.0, "d"=0.0, "underlying_def"="", "description"="A therm is one hundred thousand BTU (but depends on the definition of BTU). \n\t\t\t\tThe therm (EC) is legally defined in the Council Directive of 20 December 1979, Council of the \n\t\t\t\tEuropean Communities (now the European Union, EU). \n\t\t\t\tIt is based on the International Table Btu.\n\t\t\t"}, {"symbol"="therm[UK]", "name"="United Kingdom therm", "dimension"="L2M/T2", "is_si_unit"=TRUE, "category"="atom", "base_unit"="J", "conversion_reference"="UK-1995", "is_exact"=TRUE, "a"=0.0, "b"=105505585.257348, "c"=1.0, "d"=0.0, "underlying_def"="1E5 Btu[UK]", "description"="A therm is one hundred thousand BTU (but depends on the definition of BTU)."}, {"symbol"="therm[US]", "name"="United States therm", "dimension"="L2M/T2", "is_si_unit"=TRUE, "category"="atom", "base_unit"="J", "conversion_reference"="NIST-SI", "is_exact"=TRUE, "a"=0.0, "b"=105480400.0, "c"=1.0, "d"=0.0, "underlying_def"="", "description"="A therm is one hundred thousand BTU (but depends on the definition of BTU). \n\t\t\t\tThe therm (US) is legally defined in the Federal Register of July 27, 1968. \n\t\t\t\tAlthough the therm (EC), which is based on the International Table Btu, is frequently used by \n\t\t\t\tengineers in the United States, the therm (US) is the legal unit used by the U.S. \n\t\t\t\tnatural gas industry.\n\t\t\t"}, {"symbol"="N.m", "name"="newton metre", "dimension"="L2M/T2", "is_si_unit"=TRUE, "category"="derived", "base_unit"="", "conversion_reference"="", "is_exact"=FALSE, "a"=0.0, "b"=0.0, "c"=0.0, "d"=0.0, "underlying_def"="J", "description"=""}, {"symbol"="1E6 Btu[IT]", "name"="million BTU", "dimension"="L2M/T2", "is_si_unit"=TRUE, "category"="derived", "base_unit"="J", "conversion_reference"="DERIVED", "is_exact"=TRUE, "a"=0.0, "b"=1055055852.62, "c"=1.0, "d"=0.0, "underlying_def"="", "description"=""}, {"symbol"="GW.h", "name"="gigawatt hour", "dimension"="L2M/T2", "is_si_unit"=TRUE, "category"="derived", "base_unit"="J", "conversion_reference"="DERIVED", "is_exact"=TRUE, "a"=0.0, "b"=3600000000000.0, "c"=1.0, "d"=0.0, "underlying_def"="", "description"=""}, {"symbol"="hp.h", "name"="horsepower hour", "dimension"="L2M/T2", "is_si_unit"=TRUE, "category"="derived", "base_unit"="J", "conversion_reference"="DERIVED", "is_exact"=TRUE, "a"=0.0, 
